vi "sub_cmdbuf_fgv.vi"(7 "cmd":enum16{"ini", "add", "use", "check"}(ring), 11 "cmd":string) -> (2 "data":bool, 3 "element":string)   [LabVIEW 2018]
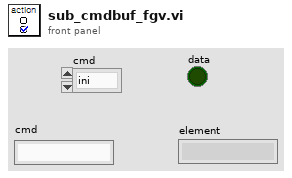
[diagram p1: front panel]
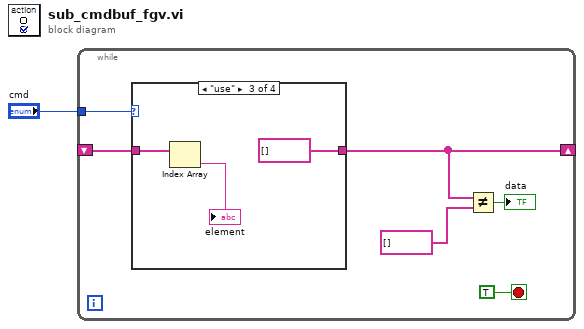
[diagram p0: block diagram]
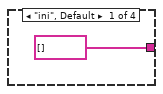
[diagram p2: hidden frame]
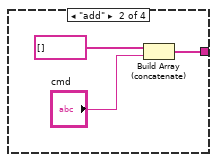
[diagram p3: hidden frame]
diagram:
  n1 = while {
    tunnel: "cmd" -> [w6]
    shift-right: [w4] -> _
    shift-left: _ -> [w5]
    stop <- TRUE stop-if-true
    n2 = case shown="\"use\"" w6 {
      tunnel: w5 -> [_ _ w14 w15]
      tunnel: [string[] [] w10 string[] [] w15] -> w4
      frame "ini", Default {
      }
      frame "add" {
        n3 = Build Array (concatenate)(string[] [], "cmd") -> (w10:string[])
      }
      frame "use" {
        n4 = Index Array(array=w14) -> (element=→"element":string)  [unwired: 1 in]
      }
      frame "check" {
      }
    }
    n5 = Not Equal?(x=w4, y=string[] []) -> (x != y?=→"data":bool)
  }
